vi "egg-signal-simulation.vi"() -> ()   [LabVIEW 2026]
uses:
  <vilib>/express/express analysis/Spectral/Block/exnSpectralBlock spectral measurements peak poly.vi
  <vilib>/express/express analysis/Spectral/Block/exnSpectralBlock spectral measurements peak WFM.vi
  <vilib>/express/express analysis/Spectral/XNode/ExpressSpectralMeasurementsBlockNode.xnode
panel:
  out "Rhythm Type":string
  out "Frequencies":dbl[](array[numeric])
  out "Amplitude":dbl[](array[numeric])
  in  "Basic Rhythm Amplitude — Min":dbl(knob) scale=150.0..300.0
  in  "Basic Rhythm Frequency — Min":dbl(knob) scale=0.02..0.08
  in  "Basic Rhythm Amplitude — Max":dbl(knob) scale=150.0..300.0
  in  "Basic Rhythm Frequency — Max":dbl(knob) scale=0.02..0.08
  out "Frequency-Domain Signal Display":cluster{"f0":dbl, "df":dbl, "magnitude":dbl[]}(graph)
  in  "Signal Generation":bool
  in  "Respiratory Disturbance Amplitude — Min":dbl(knob) scale=10.0..50.0
  in  "Respiratory Disturbance Amplitude — Max":dbl(knob) scale=10.0..50.0
  in  "Respiratory Disturbance Frequency — Min":dbl(knob) scale=0.15..0.25
  in  "Respiratory Disturbance Frequency — Max":dbl(knob) scale=0.15..0.25
  in  "Start":bool
  out "Signal Display":dbl(graph)
  in  "Sampling Frequency":dbl
  # "(the first amplitude and frequency values represent respiratory disturbances, the next two represent harmonics, and the remaining values represent the basic rhythm)"
  # "frekvencija je u Hz, a amplitude su u µV"
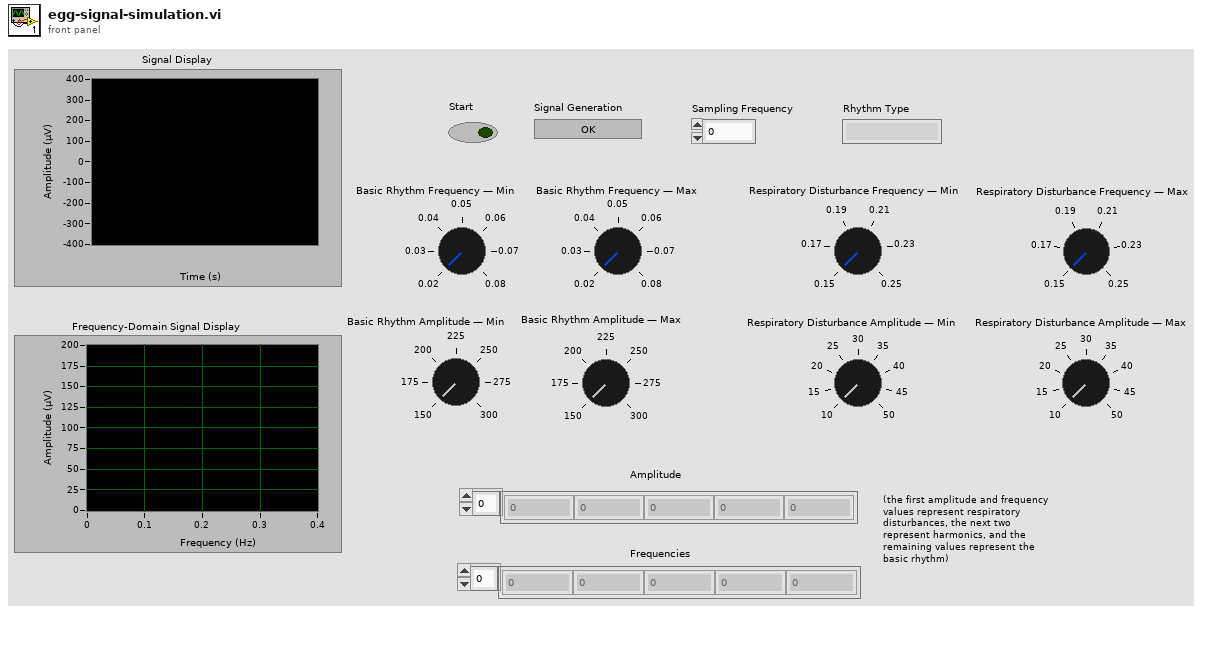
[diagram p1: front panel]
types:
  T1 = cluster{"averaging mode":u16, "weighting mode":u16, "number of averages":u32}
  T2 = cluster{"dB On (F)":bool, "unwrap phase (F)":bool, "convert to degree (F)":bool}
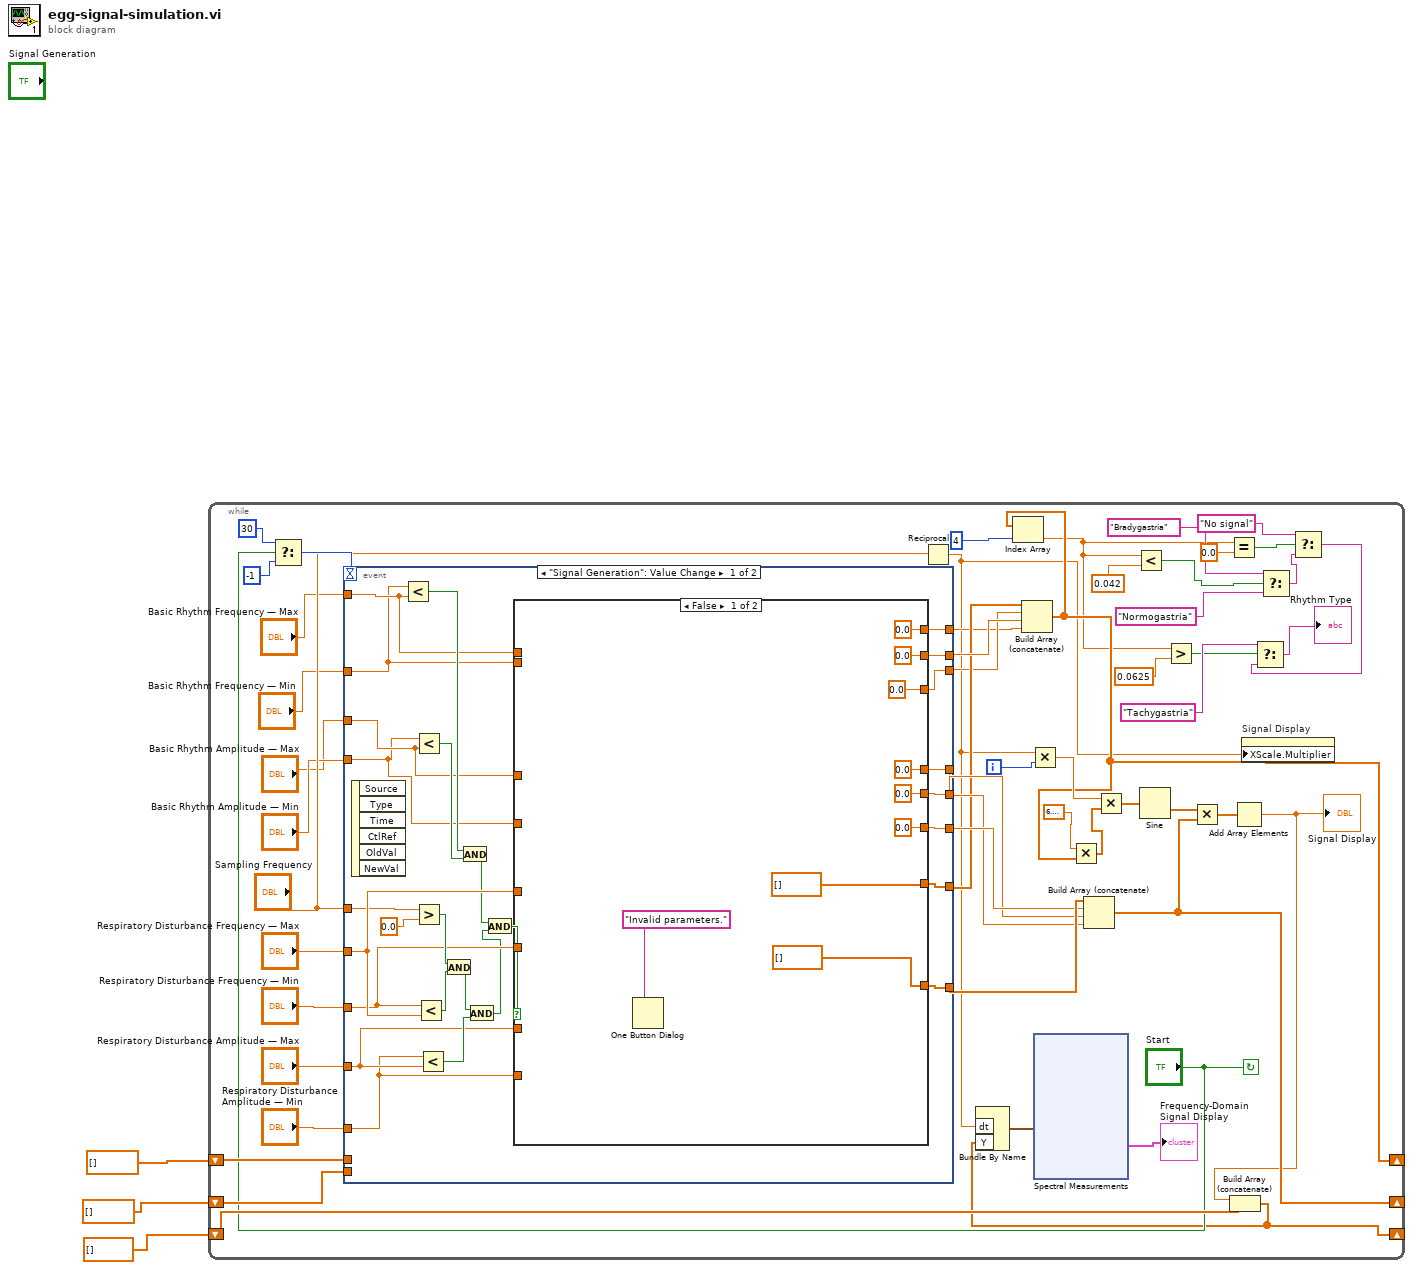
[diagram p0: block diagram]
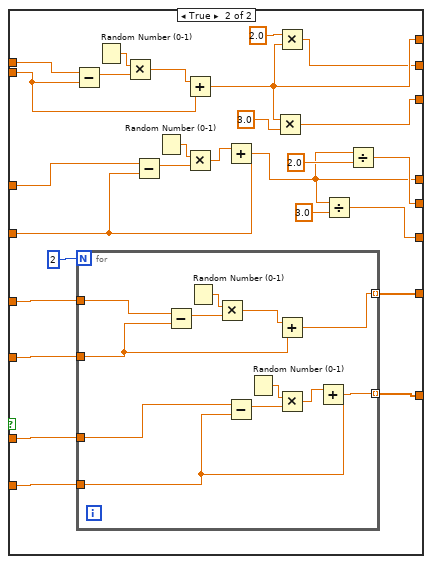
[diagram p2: hidden frame]
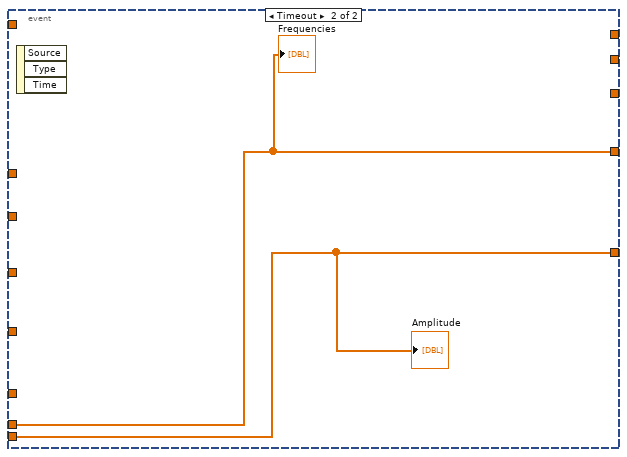
[diagram p3: hidden frame]
diagram:
  n1 = while {
    shift-right: [w23] -> _
    shift-left: dbl[] [] -> [w47]
    shift-right: [w31] -> _
    shift-left: dbl[] [] -> [w46]
    shift-right: [w14] -> _
    shift-left: dbl[] [] -> [w45]
    i -> [w44]
    stop <- "Start" continue-if-true
    n2 = Select(t=30, s="Start", f=-1) -> (s? t:f=w40:i32)
    n3 = event shown="[0] \"Signal Generation\": Value Change" {
      selector: _ -> [_ _]
      dyn-events: _ -> [_ _]
      timeout: w40 -> [_ _]
      tunnel: [w89 w143] -> w30
      tunnel: "Respiratory Disturbance Frequency — Max" -> [w88 _]
      tunnel: "Respiratory Disturbance Frequency — Min" -> [w87 _]
      tunnel: "Respiratory Disturbance Amplitude — Max" -> [w86 _]
      tunnel: "Respiratory Disturbance Amplitude — Min" -> [w85 _]
      tunnel: "Sampling Frequency" -> [w84 _]
      tunnel: w46 -> [_ w143]
      tunnel: w45 -> [_ w142]
      tunnel: [w83 w142] -> w25
      tunnel: "Basic Rhythm Frequency — Max" -> [w76 _]
      tunnel: "Basic Rhythm Frequency — Min" -> [w75 _]
      tunnel: "Basic Rhythm Amplitude — Min" -> [w73 _]
      tunnel: "Basic Rhythm Amplitude — Max" -> [w74 _]
      tunnel: [w72 _] -> w24
      tunnel: [w71 _] -> w27
      tunnel: [w70 _] -> w13
      tunnel: [w69 _] -> w26
      tunnel: [w68 _] -> w28
      tunnel: [w67 _] -> w29
      event "Signal Generation": Value Change {
        n4 = event-data() -> ()  [unwired: 1 in, 6 out]
        n5 = Less?(x=w75, y=w76) -> (x < y?=w77:bool)
        n6 = Less?(x=w73, y=w74) -> (x < y?=w78:bool)
        n7 = Greater?(x=w84, y=0.0) -> (0:w93:bool)
        n8 = Less?(x=w87, y=w88) -> (x < y?=w92:bool)
        n9 = Less?(x=w85, y=w86) -> (x < y?=w90:bool)
        n10 = And(x=w93, y=w92) -> (x .and. y?=w91:bool)
        n11 = And(x=w77, y=w78) -> (x .and. y?=w80:bool)
        n12 = And(x=w91, y=w90) -> (x .and. y?=w81:bool)
        n13 = And(x=w80, y=w81) -> (x .and. y?=w79:bool)
        n14 = case shown="False" w79 {
          tunnel: w88 -> [_ w128]
          tunnel: w87 -> [_ w127]
          tunnel: w86 -> [_ w126]
          tunnel: w85 -> [_ w125]
          tunnel: [dbl[] [] w124] -> w89
          tunnel: [dbl[] [] w123] -> w83
          tunnel: w76 -> [_ w116]
          tunnel: w75 -> [_ w115]
          tunnel: w74 -> [_ w114]
          tunnel: w73 -> [_ w113]
          tunnel: [0.0 w103] -> w72
          tunnel: [0.0 w107] -> w71
          tunnel: [0.0 w105] -> w70
          tunnel: [0.0 w104] -> w69
          tunnel: [0.0 w109] -> w68
          tunnel: [0.0 w108] -> w67
          frame False {
            n15 = One Button Dialog(message="Invalid parameters.") -> ()  [unwired: 1 in, 1 out]
          }
          frame True {
            n16 = Subtract(x=w116, y=w115) -> (x-y=w121:dbl)
            n17 = for {
              N: 2 -> [_]
              tunnel: w128 -> [w134]
              tunnel: w127 -> [w133]
              tunnel: w126 -> [w132]
              tunnel: w125 -> [w131]
              tunnel: [w130] -> w124 mode=indexing
              tunnel: [w139] -> w123 mode=indexing
              n18 = Subtract(x=w134, y=w133) -> (x-y=w140:dbl)
              n19 = Random Number (0-1)() -> (number: 0 to 1=w141:dbl)
              n20 = Multiply(x=w141, y=w140) -> (x*y=w138:dbl)
              n21 = Subtract(x=w132, y=w131) -> (x-y=w136:dbl)
              n22 = Random Number (0-1)() -> (number: 0 to 1=w137:dbl)
              n23 = Add(x=w138, y=w133) -> (x+y=w139:dbl)
              n24 = Multiply(x=w137, y=w136) -> (x*y=w135:dbl)
              n25 = Add(x=w135, y=w131) -> (x+y=w130:dbl)
            }
            n26 = Random Number (0-1)() -> (number: 0 to 1=w122:dbl)
            n27 = Multiply(x=w122, y=w121) -> (x*y=w120:dbl)
            n28 = Subtract(x=w114, y=w113) -> (x-y=w118:dbl)
            n29 = Random Number (0-1)() -> (number: 0 to 1=w119:dbl)
            n30 = Add(x=w120, y=w115) -> (x+y=w105:dbl)
            n31 = Multiply(x=w119, y=w118) -> (x*y=w117:dbl)
            n32 = Add(x=w117, y=w113) -> (x+y=w107:dbl)
            n33 = Multiply(x=w105, y=3.0 ("x")) -> (x*y=w103:dbl)
            n34 = Multiply(x=2.0, y=w105) -> (x*y=w104:dbl)
            n35 = Divide(x=w107, y=3.0) -> (x/y=w108:dbl)
            n36 = Divide(x=w107, y=2.0) -> (x/y=w109:dbl)
          }
        }
      }
      event Timeout {
        n37 = event-data() -> ()  [unwired: 1 in, 3 out]
        "Amplitude" <- w143
        "Frequencies" <- w142
      }
    }
    n38 = Reciprocal(x="Sampling Frequency") -> (1/x=w11:dbl)
    n39 = Build Array (concatenate)(w25, w24, w26, w13) -> (w14:dbl[])
    n40 = Index Array(array=w14, index=4) -> (element=w9:dbl)
    n41 = Multiply(x=w11, y=w44) -> (x*y=w36:dbl)
    n42 = Multiply(x=6.283185307179586, y=w14) -> (x*y=w50:dbl[])
    n43 = Build Array (concatenate)(w30, w29, w28, w27) -> (w31:dbl[])
    n44 = Multiply(x=w36, y=w50) -> (x*y=w49:dbl[])
    n45 = Less?(x=w9, y=0.042) -> (x < y?=w10:bool)
    n46 = Sine(x=w49) -> (sin(x)=w56:dbl[])
    n47 = Greater?(x=w9, y=0.0625) -> (0:w17:bool)
    n48 = Multiply(x=w56, y=w31) -> (x*y=w48:dbl[])
    n49 = Equal?(x=w9, y=0.0) -> (x = y?=w7:bool)
    n50 = Add Array Elements(numeric array=w48) -> (sum=w12:dbl)
    "Signal Display" <- w12
    n51 = Build Array (concatenate)(w12, w47) -> (w23:dbl[])
    n52 = Bundle By Name("dt"=w11, "Y"=w23) -> (w42:waveform(dbl))  [unwired: 1 in]
    n53 = xnode "Spectral Measurements"("Signals"=w42) -> ("FFT - (Peak)"=→"Frequency-Domain Signal Display":cluster{"f0":dbl, "df":dbl, "magnitude":dbl[]})  [unwired: 1 in, 2 out]
    n54 = property on="Signal Display" class="WFChart (strict)"("XScale.Multiplier"=w11) -> ()  [unwired: 2 in, 2 out]
    n55 = Select(t="Bradygastria" ("Stanje"), s=w10, f="Normogastria" ("Stanje")) -> (s? t:f=w5:string)
    n56 = Select(t="No signal" ("Stanje"), s=w7, f=w5) -> (s? t:f=w4:string)
    n57 = Select(t="Tachygastria" ("Stanje"), s=w17, f=w4) -> (s? t:f=→"Rhythm Type":string)
  }
